vi "Data Check.vi"(6 "Spec List":cluster{"Lower":dbl, "Upper":dbl}[](array[cluster]), 8 "error in (no error)":errorcluster, 10 "Test Spec":T1={"PSU "={"Lower"=0.0002, "Upper"=1.0}, "Sensitivity"={"Lower"=0.2121, "Upper"=0.4243}, "THD"={"Lower"=1.0, "Upper"=0.0}}, 11 "Data":T2) -> (0 "error out":errorcluster, 2 "All Result":bool)   [LabVIEW 2018]
uses:
  Controls/DataType.ctl
panel:
  out "Sensitivity Result 2":bool
  out "THD Result 2":bool
  out "Freq Result 2":bool
  out "Freq Result 1":bool
  out "THD Result 1":bool
  out "Sensitivity Result 1":bool
  out "PSU Result":bool
  # "Spec comparison"
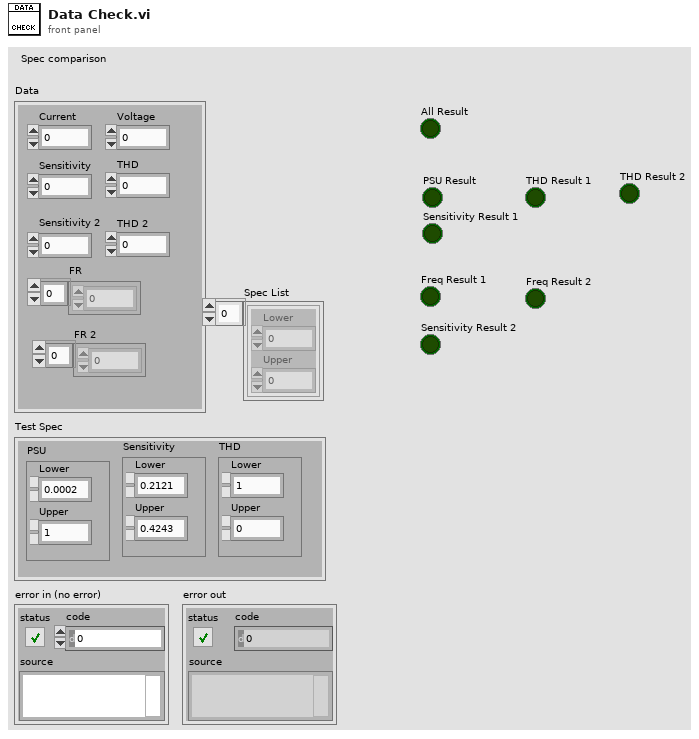
[diagram p1: front panel]
types:
  T1 = cluster{"PSU ":cluster{"Lower":dbl, "Upper":dbl}, "Sensitivity":cluster{"Lower":dbl, "Upper":dbl}, "THD":cluster{"Lower":dbl, "Upper":dbl}}
  T2 = typedef "DataType.ctl" = cluster{"Current":dbl, "Voltage":dbl, "Sensitivity":dbl, "THD":dbl, "FR":dbl[], "Sensitivity 2":dbl, "THD 2":dbl, "FR 2":dbl[]}
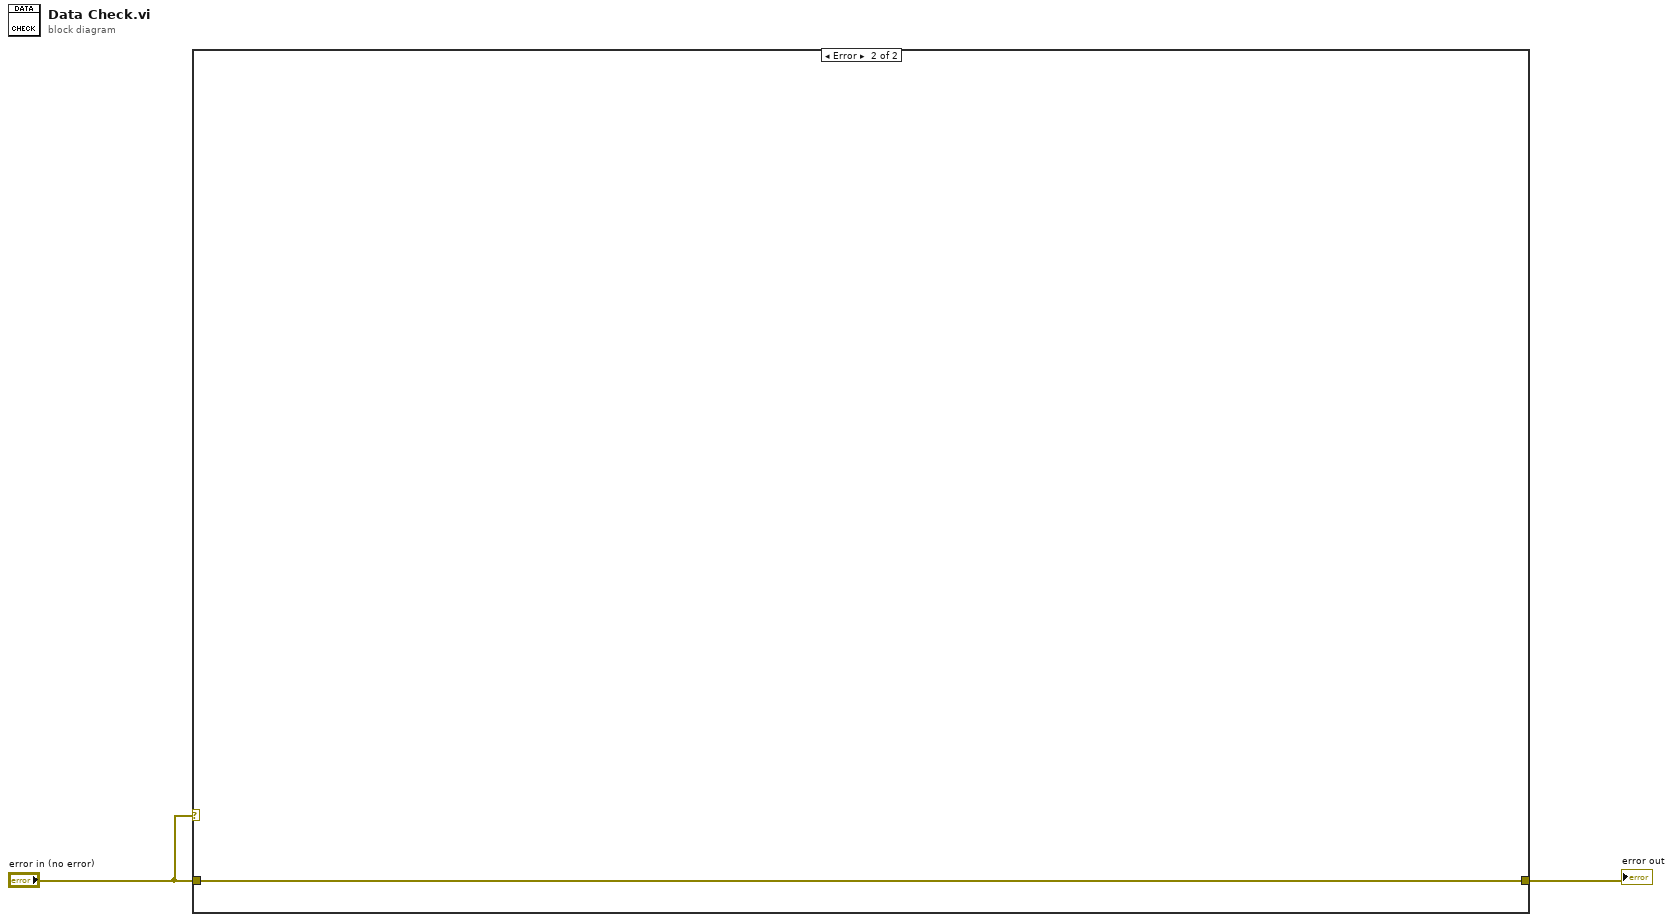
[diagram p0: block diagram]
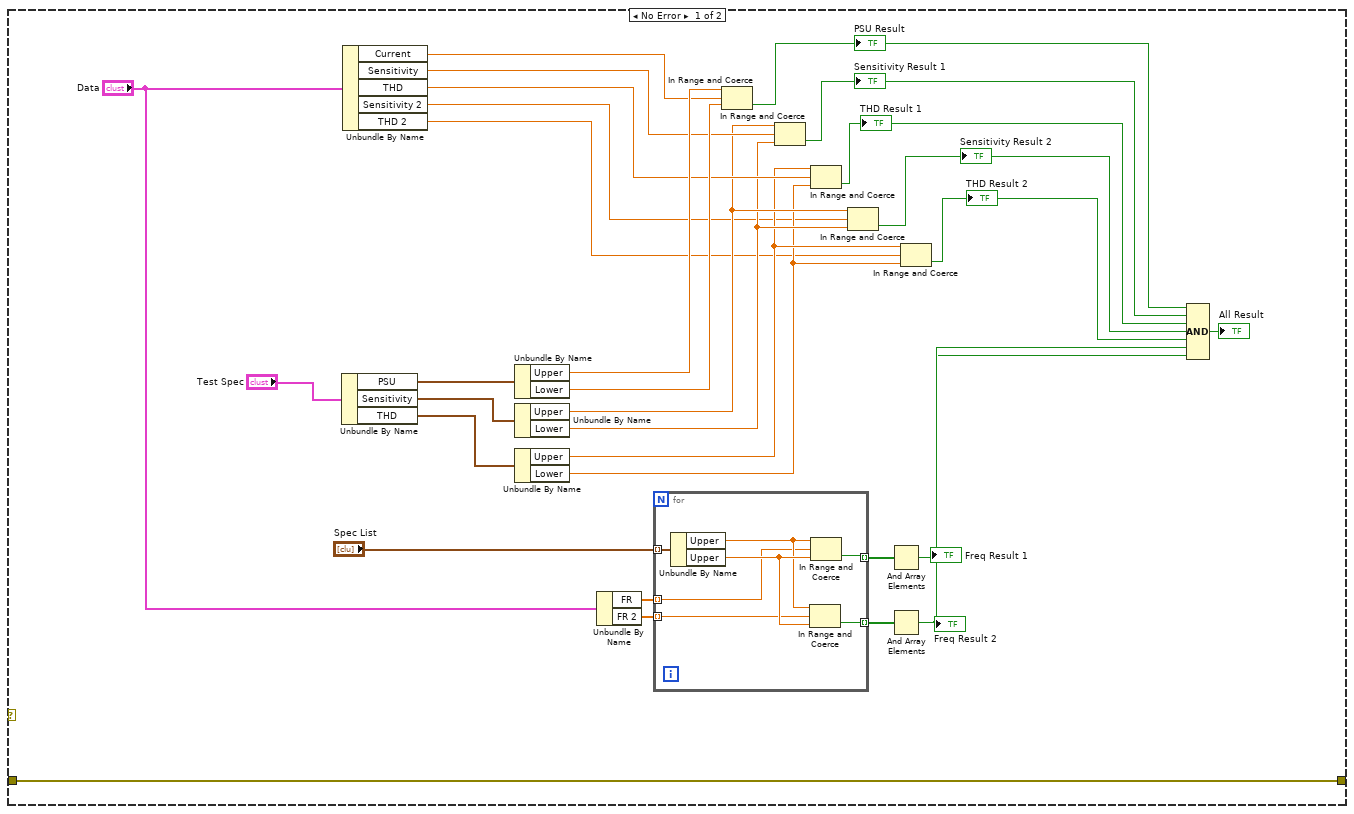
[diagram p2: hidden frame]
diagram:
  n1 = case shown="Error" "error in (no error)" {
    tunnel: "error in (no error)" -> [w3 w40]
    tunnel: [w3 w40] -> w2
    frame No Error {
      n2 = Unbundle By Name("Test Spec") -> ("PSU"=w28:cluster{"Lower":dbl, "Upper":dbl}, "Sensitivity"=w27:cluster{"Lower":dbl, "Upper":dbl}, "THD"=w26:cluster{"Lower":dbl, "Upper":dbl})
      n3 = Unbundle By Name("Data") -> ("Current"=w30:dbl, "Sensitivity"=w24:dbl, "THD"=w23:dbl, "Sensitivity 2"=w18:dbl, "THD 2"=w17:dbl)
      n4 = Unbundle By Name(w28) -> ("Upper"=w32:dbl, "Lower"=w31:dbl)
      n5 = Unbundle By Name(w27) -> ("Upper"=w22:dbl, "Lower"=w21:dbl)
      n6 = Unbundle By Name(w26) -> ("Upper"=w20:dbl, "Lower"=w19:dbl)
      n7 = Unbundle By Name("Data") -> ("FR"=w15:dbl[], "FR 2"=w14:dbl[])
      n8 = for {
        tunnel: "Spec List" -> [w39] mode=indexing
        tunnel: w15 -> [w36] mode=indexing
        tunnel: w14 -> [w35] mode=indexing
        tunnel: [w34] -> w13 mode=indexing
        tunnel: [w33] -> w12 mode=indexing
        n9 = Unbundle By Name(w39) -> ("Upper"=w37:dbl, "Upper"=w38:dbl)
        n10 = In Range and Coerce(upper limit=w37, x=w35, lower limit=w38) -> (In Range?=w33:bool)  [unwired: 1 out]
        n11 = In Range and Coerce(upper limit=w37, x=w36, lower limit=w38) -> (In Range?=w34:bool)  [unwired: 1 out]
      }
      n12 = In Range and Coerce(upper limit=w32, x=w30, lower limit=w31) -> (In Range?=w11:bool)  [unwired: 1 out]
      "PSU Result" <- w11
      n13 = In Range and Coerce(upper limit=w22, x=w24, lower limit=w21) -> (In Range?=w10:bool)  [unwired: 1 out]
      "Sensitivity Result 1" <- w10
      n14 = In Range and Coerce(upper limit=w20, x=w23, lower limit=w19) -> (In Range?=w9:bool)  [unwired: 1 out]
      "THD Result 1" <- w9
      n15 = In Range and Coerce(upper limit=w22, x=w18, lower limit=w21) -> (In Range?=w8:bool)  [unwired: 1 out]
      "Sensitivity Result 2" <- w8
      n16 = And Array Elements(Boolean array=w13) -> (logical AND=w6:bool)
      "Freq Result 1" <- w6
      n17 = And Array Elements(Boolean array=w12) -> (logical AND=w5:bool)
      "Freq Result 2" <- w5
      n18 = In Range and Coerce(upper limit=w20, x=w17, lower limit=w19) -> (In Range?=w7:bool)  [unwired: 1 out]
      "THD Result 2" <- w7
      n19 = Compound Arithmetic op=AND(w11, w10, w9, w8, w7, w6, w5) -> (→"All Result":bool)
    }
    frame Error {
    }
  }
  "error out" <- w2
